vi "Close COM Port.vi"() -> ()   [LabVIEW 2018]
panel:
  out "find list":string[](array[string])
  in  "VISA resource name":refnum<visa-resource-name>="COM10"
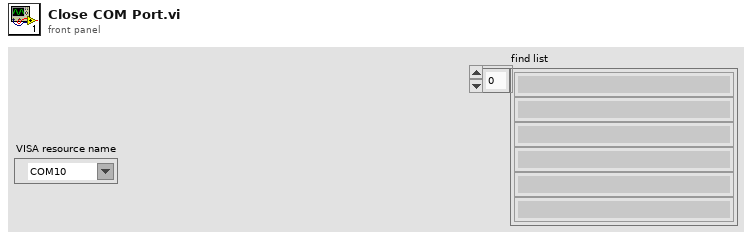
[diagram p1: front panel]
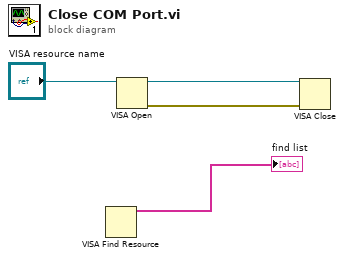
[diagram p0: block diagram]
diagram:
  n1 = VISA Find Resource() -> (3:→"find list":string[])  [unwired: 3 in, 2 out]
  n2 = VISA Open(VISA resource name="VISA resource name") -> (VISA resource name=w4:refnum<visa-resource-name>, error out=w3:errorcluster)  [unwired: 4 in]
  n3 = VISA Close(VISA resource name=w4, error in (no error)=w3) -> ()  [unwired: 1 out]
